vi "Read_register_cmd.vi"(7 "Fifo-mode En":bool, 8 "Arty-7 Error In":errorcluster, 9 "Words_to_read":u16, 10 "RdReg Addr":u8 format="%b", 11 "Arty-7 VISA In":refnum<visa-resource-name>) -> (0 "Arty-7 Error out":errorcluster, 1 "RdReg Status":string, 2 "RdReg Done":bool, 3 "Arty-7 VISA out":refnum<visa-resource-name>, 4 "RdReg Data":u8[](array[numeric]))   [LabVIEW 2019]
uses:
  <vilib>/Utility/error.llb/DialogType.ctl
  Board_Global_Var.vi
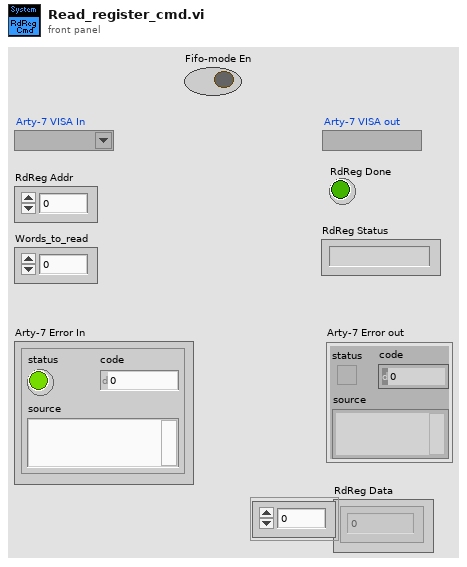
[diagram p1: front panel]
types:
  T1 = typedef "DialogType.ctl" = u16
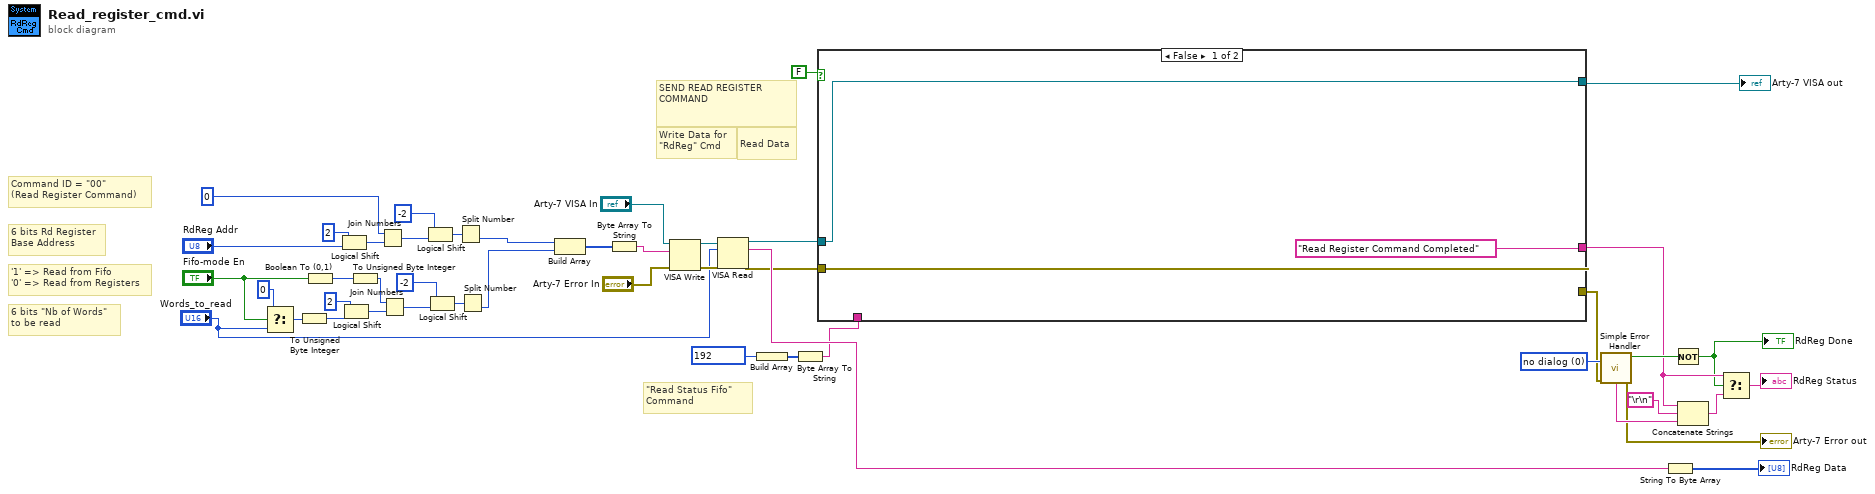
[diagram p0: block diagram]
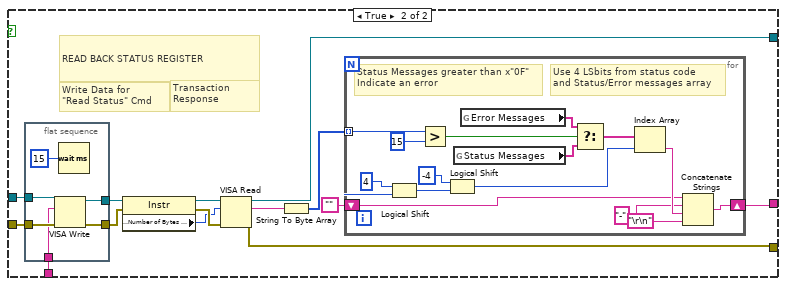
[diagram p2: hidden frame]
diagram:
  w18 = T1 0 items=["no dialog", "OK message", "continue or stop message", "OK message + warnings", "continue/stop + warnings"] ("type of dialog (OK msg:1)")
  # "\"Read Status Fifo\" \nCommand"
  # "SEND READ REGISTER\nCOMMAND"
  # "Read Data"
  # "Write Data for \n\"RdReg\" Cmd"
  # "'1' => Read from Fifo\n'0' => Read from Registers"
  # "6 bits \"Nb of Words\"\nto be read"
  # "6 bits Rd Register \nBase Address"
  # "Command ID = \"00\" \n(Read Register Command)"
  n1 = Select(t=u8 0, s="Fifo-mode En", f="Words_to_read") -> (s? t:f=w5:u16)
  n2 = To Unsigned Byte Integer(number=w5) -> (unsigned 8bit integer=w44:u8)
  n3 = Boolean To (0,1)(Boolean="Fifo-mode En") -> (0, 1=w36:i16)
  n4 = Logical Shift(y=i16 2, x="RdReg Addr") -> (x << y=w25:u8)
  n5 = Logical Shift(y=i16 2, x=w44) -> (x << y=w32:u8)
  n6 = To Unsigned Byte Integer(number=w36) -> (unsigned 8bit integer=w37:u8)
  n7 = Join Numbers(hi=u8 0, lo=w25) -> ((hi.lo)=w24:u16)
  n8 = Join Numbers(hi=w37, lo=w32) -> ((hi.lo)=w33:u16)
  n9 = Logical Shift(y=i16 -2, x=w24) -> (x << y=w28:u16)
  n10 = Logical Shift(y=i16 -2, x=w33) -> (x << y=w30:u16)
  n11 = Split Number(x=w28) -> (lo(x)=w29:u8)  [unwired: 1 out]
  n12 = Split Number(x=w30) -> (lo(x)=w35:u8)  [unwired: 1 out]
  n13 = Build Array(w29, w35) -> (w39:u8[])
  n14 = Byte Array To String(unsigned byte array=w39) -> (string=w38:string)
  n15 = VISA Write(VISA resource name="Arty-7 VISA In", write buffer=w38, error in (no error)="Arty-7 Error In") -> (VISA resource name out=w43:refnum<visa-resource-name>, error out=w42:errorcluster)  [unwired: 1 out]
  n16 = VISA Read(VISA resource name=w43, byte count="Words_to_read", error in (no error)=w42) -> (VISA resource name out=w12:refnum<visa-resource-name>, read buffer=w41:string, error out=w11:errorcluster)  [unwired: 1 out]
  n17 = Build Array(u8 192) -> (w46:u8[])
  n18 = Byte Array To String(unsigned byte array=w46) -> (string=w10:string)
  n19 = case shown="False" FALSE {
    tunnel: [w48 w63] -> w9
    tunnel: [w47 w62] -> w17
    tunnel: ["Read Register Command Completed" w60] -> w16
    tunnel: w12 -> [w48 w52]
    tunnel: w11 -> [w47 w51]
    tunnel: w10 -> [_ w50]
    frame False {
    }
    frame True {
      # "READ BACK STATUS REGISTER"
      # "Write Data for \n\"Read Status\" Cmd"
      # "Transaction \nResponse"
      n20 = flat-sequence {
        tunnel: [w69] -> w59
        tunnel: [w68] -> w58
        tunnel: w52 -> [w66]
        tunnel: w51 -> [w65]
        tunnel: w50 -> [w64]
        frame #0 {
          n21 = VISA Write(VISA resource name=w66, write buffer=w64, error in (no error)=w65) -> (VISA resource name out=w69:refnum<visa-resource-name>, error out=w68:errorcluster)  [unwired: 1 out]
          n22 = Wait (ms)(milliseconds to wait=u32 15) -> ()  [unwired: 1 out]
        }
      }
      n23 = property class="Instr"(reference=w59, error in=w58) -> (reference out=w57:refnum<visa-resource-name>, error out=w56:errorcluster, "Serial Settings:Number of Bytes at Serial Port"=w55:u32)
      n24 = VISA Read(VISA resource name=w57, byte count=w55, error in (no error)=w56) -> (VISA resource name out=w63:refnum<visa-resource-name>, read buffer=w61:string, error out=w62:errorcluster)  [unwired: 1 out]
      n25 = String To Byte Array(string=w61) -> (unsigned byte array=w54:u8[])
      n26 = for {
        tunnel: w54 -> [w74] mode=indexing
        shift-right: [w73] -> w60
        shift-left: "" -> [w72]
        # "Use 4 LSbits from status code \nand Status/Error messages array"
        # "Status Messages greater than x\"0F\"\nIndicate an error"
        n27 = Logical Shift(y=i16 4, x=w74) -> (x << y=w77:u8)
        n28 = Greater?(x=w74, y=u8 15) -> (0:w80:bool)
        n29 = Logical Shift(y=i16 -4, x=w77) -> (x << y=w78:u8)
        n30 = global read "Board_Global_Var.vi" "Status Messages"() -> (w81:string[])
        n31 = global read "Board_Global_Var.vi" "Error Messages"() -> (w82:string[])
        n32 = Select(t=w82, s=w80, f=w81) -> (s? t:f=w83:string[])
        n33 = Index Array(array=w83, index=w78) -> (element=w75:string)
        n34 = Concatenate Strings(w72, "-" ("string"), w75, "\r\n") -> (w73:string)
      }
    }
  }
  "Arty-7 VISA out" <- w9
  n35 = call <vilib>:"Simple Error Handler.vi"("type of dialog (OK msg:1)"=w18, "error in (no error)"=w17) -> ("error?"=w19:bool, "error out"=→"Arty-7 Error out":errorcluster, "message"=w14:string)  [unwired: 3 in, 2 out]
  n36 = String To Byte Array(string=w41) -> (unsigned byte array=→"RdReg Data":u8[])
  n37 = Not(x=w19) -> (.not. x?=w6:bool)
  "RdReg Done" <- w6
  n38 = Concatenate Strings(w16, "\r\n", w14) -> (w13:string)
  n39 = Select(t=w16, s=w6, f=w13) -> (s? t:f=→"RdReg Status":string)
